vi "Configure TClk.vi"(0 "session in":refnum<class "Digitizer Control.lvclass">, 1 "TClk API Control Enable":T1, 5 "error in (no error)":errorcluster) -> (14 "session out":refnum<class "Digitizer Control.lvclass">, 19 "error out":errorcluster)   [LabVIEW 2021, in "Digitizer Control.lvclass"]
doc: "Configures the signal acquisition to be controlled by the TClk API.\n\nInputs:\n\n<B>session in</B>: The device session.\n\n<B>TClk API Control Enable</B>: Selects the direction the TClk API should control. The <B>Acquisition</B> option selects the signal acquisition to be controlled by the TClk API. The start trigger should be configured on the TClk master only, using the <B>Acq Configure Start Trigger.vi</B>.\n\nOutput:\n\n<B>session out</B>: The device session passed on the <B>session in</B> input."
uses:
  Digitizer Control.lvclass
  TClk API Control Enable.ctl
  Digitizer Control.lvclass/Digitizer Control.ctl
  <instrlib>/FlexRIO/API/Host/v1/NI FlexRIO/API/Get Property Reference - Fpga Small.vi
  <resource>/objmgr/niflexrioapiStream.rc
  <instrlib>/FlexRIO/API/Host/v1/NI FlexRIO API v1.lvlib
  <resource>/objmgr/niflexrioapi.rc
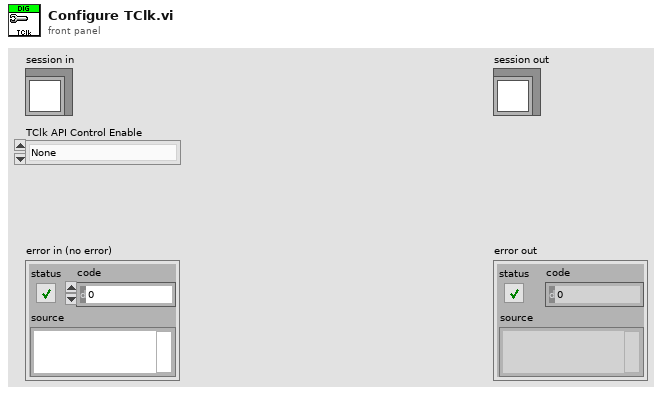
[diagram p1: front panel]
types:
  T1 = typedef "Digitizer Control.lvclass/TClk API Control Enable.ctl" = enum16{"None", "Acquisition"}
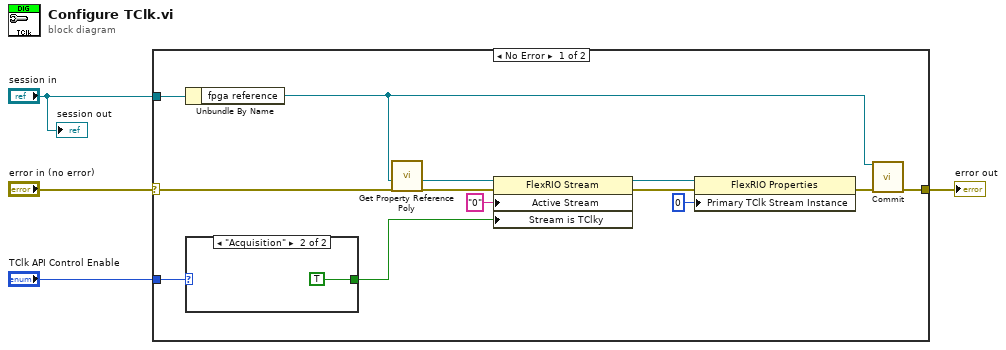
[diagram p0: block diagram]
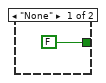
[diagram p2: hidden frame]
diagram:
  n1 = case shown="No Error" "error in (no error)" {
    selector: "error in (no error)" -> [w5 w20]
    tunnel: "session in" -> [w11 _]
    tunnel: [w9 w20] -> w3
    tunnel: "TClk API Control Enable" -> [w13 _]
    frame No Error {
      n2 = Unbundle By Name(w11) -> ("fpga reference"=w6:refnum<k20>)
      n3 = case shown="\"Acquisition\"" w13 {
        tunnel: [FALSE TRUE] -> w12
        frame "None" {
        }
        frame "Acquisition" {
        }
      }
      n4 = call-poly <instrlib>:"Get Property Reference Poly.vi"("error in (no error)"=w5, "fpga interface in"=w6) -> ("error out"=w14:errorcluster, "property reference"=w15:refnum<k20>)  [unwired: 4 in, 1 out]
      n5 = property class="FlexRIO Stream"(reference=w15, error in=w14, "Active Stream"="0", "Stream is TClky"=w12) -> (reference out=w16:refnum<k20>, error out=w17:errorcluster)
      n6 = property class="FlexRIO Properties"(reference=w16, error in=w17, "Primary TClk Stream Instance"=0 ("Device:Primary TClk Stream Instance")) -> (error out=w10:errorcluster)  [unwired: 1 out]
      n7 = call <instrlib>:"Commit.vi"("fpga interface in"=w6, "error in"=w10) -> ("error out"=w9:errorcluster)  [unwired: 12 in, 1 out]
    }
    frame Error {
    }
  }
  "error out" <- w3
  "session out" <- "session in"
